vi "Write Verify Server.vi"(8 "error in (no error)":errorcluster, 10 "Verify Server":bool, 11 "AWS Core in":refnum<class "HTTP Request.lvclass">) -> (0 "error out":errorcluster, 3 "AWS Core out":refnum<class "HTTP Request.lvclass">)   [LabVIEW 2015, in "NI_AWS_Core.lvlib" / "HTTP Request.lvclass"]
uses:
  HTTP Request.lvclass
  HTTP Request.lvclass/HTTP Request.ctl
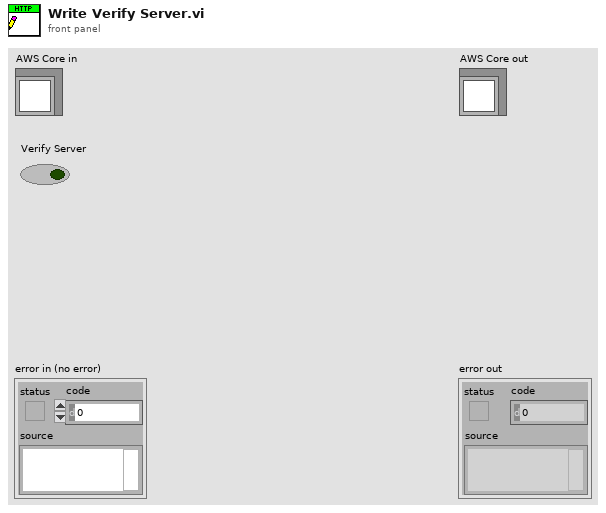
[diagram p1: front panel]
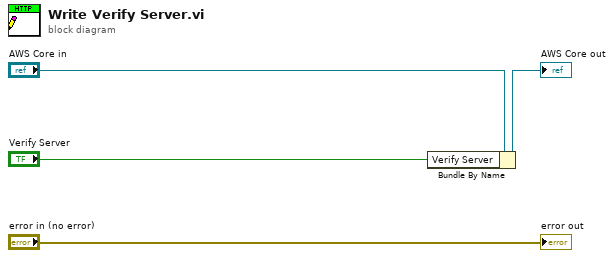
[diagram p0: block diagram]
diagram:
  n1 = Bundle By Name(cluster="AWS Core in", "Verify Server"="Verify Server") -> (→"AWS Core out":refnum<class "HTTP Request.lvclass">)
  "error out" <- "error in (no error)"
